vi "_modifyResultsStatus.vi"(11 "Current Results In":string[][](table) caption="08/08/2016 14:14:26") -> (3 "Current Results Out":string[][](table) caption="08/08/2016 14:14:26")   [LabVIEW 2015]
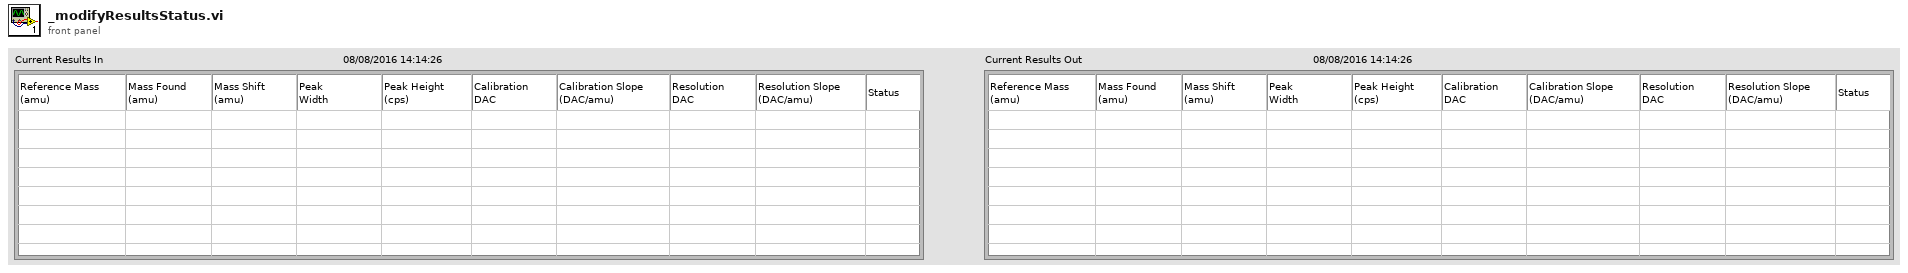
[diagram p1: front panel]
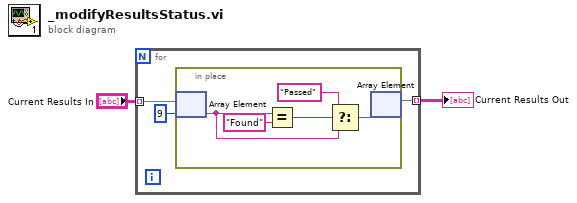
[diagram p0: block diagram]
diagram:
  n1 = for {
    tunnel: "Current Results In" -> [w5] mode=indexing
    tunnel: [w4] -> w1 mode=indexing
    n2 = in-place {
      n3 = in-place-array #1(w5, 9) -> (w6:string)
      n4 = Equal?(x=w6, y="Found") -> (x = y?=w9:bool)
      n5 = Select(t="Passed" ("y"), s=w9, f=w6) -> (s? t:f=w7:string)
      n6 = in-place-array #1(w7) -> (w4:string[])  [unwired: 1 out]
    }
  }
  "Current Results Out" <- w1
